vi "VI-Hacker v2.vi"(6 "Overwrite VI? (F)":bool, 8 "error in (no error)":errorcluster, 10 "Target Folder":path, 11 "VI Path":path) -> (0 "error out":errorcluster)   [LabVIEW 2020, in "VI-Hacker.lvlib"]
doc: "Unlocks a password protected VI.\n\nCreated by: Ryan Pacini (c) 2023"
uses:
  VI-Hacker.lvlib
panel:
  # "Unlock and Save Password Protected VI\nCreated by: Ryan Pacini (c) 2023"
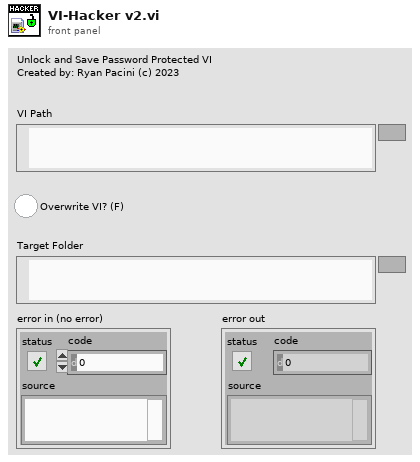
[diagram p1: front panel]
types:
  T1 = cluster{"BLOCK_INFO":cluster{"Int1":u32, "Int2":u32, "Int3":u32, "Offset":u32, "Size":u32}[]}
  T2 = cluster{"Name":string, "Idx":i32, "Data":string, "Offset":u32}
  T3 = enum16{"open", "replace", "create", "open or create", "replace or create", "replace or create with confirmation"}
  T4 = cluster{"vers":i32, "BDPW":i32, "LIBN":i32, "LVSR":i32, "BDHx":i32}
  T5 = cluster{"Version Major":u8, "Pswrd Hashes":cluster{"Pswrd (md5)":string, "Hash1 (md5)":string, "Hash2 (md5)":string}, "Owning Libs (':')":string, "Pswrd Salt (md5)":string, "Diagram (md5)":string, "BDPW Offset":u32, "New BDPW":string}
  T6 = cluster{"Pswrd (md5)":string, "Hash1 (md5)":string, "Hash2 (md5)":string}
  T7 = enum32{"invalid lock state", "Not Locked", "Locked (No Password)", "Password-protected"}
  T8 = cluster{"RSRC_Identifier":u64, "RSRC_Type":u32, "RSRC_Creator":u32, "Info_Offset":u32, "Info_Size":u32, "Data_Offset":u32, "Data_Size":u32}
  T9 = cluster{"Int1":u32, "Int2":u32, "Int3":u32, "Offset":u32, "Size":u32}
  T10 = cluster{"Int1":u32, "Int2":u32, "Int3":u32, "Offset":u32, "Size":u32}[]
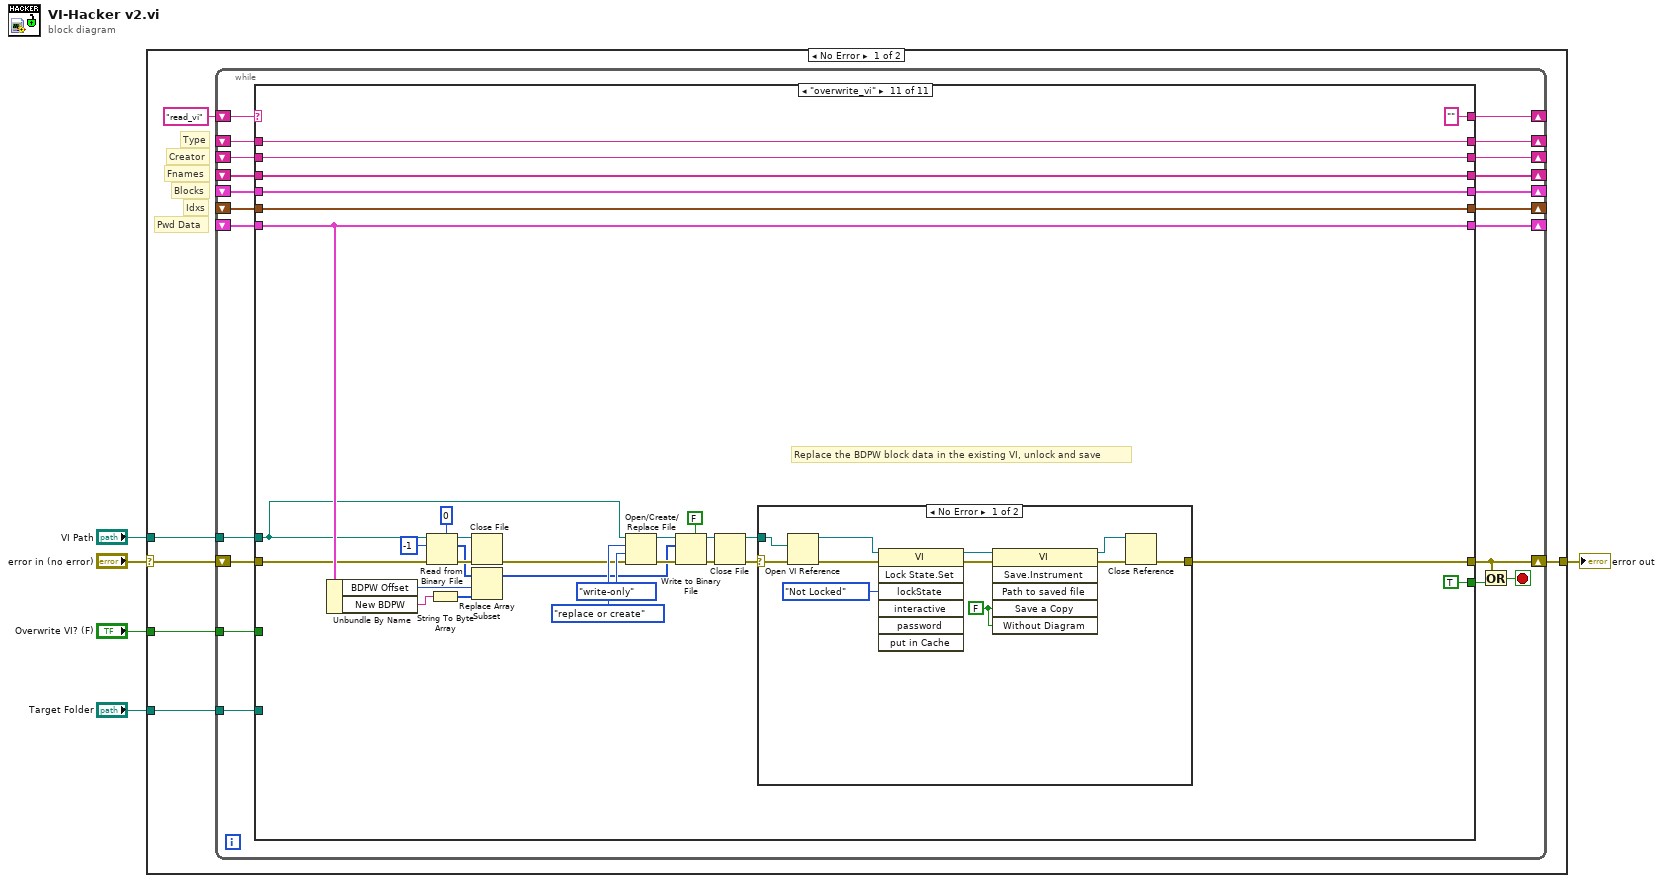
[diagram p0: block diagram]
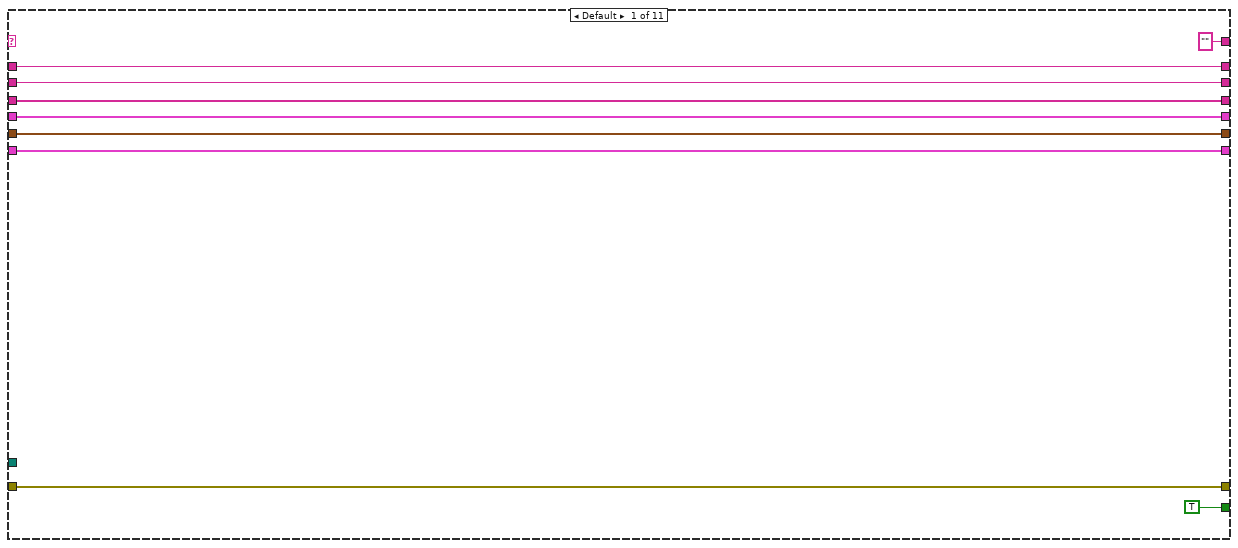
[diagram p2: hidden frame]
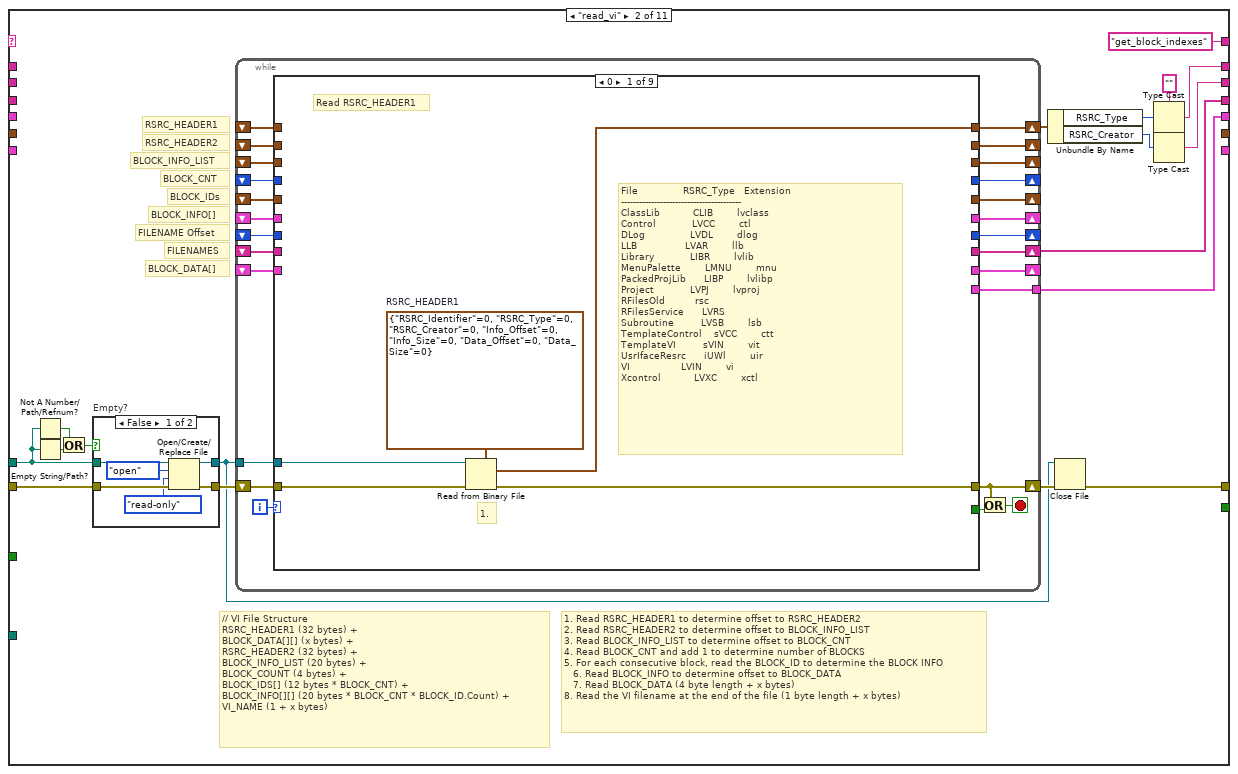
[diagram p3: hidden frame]
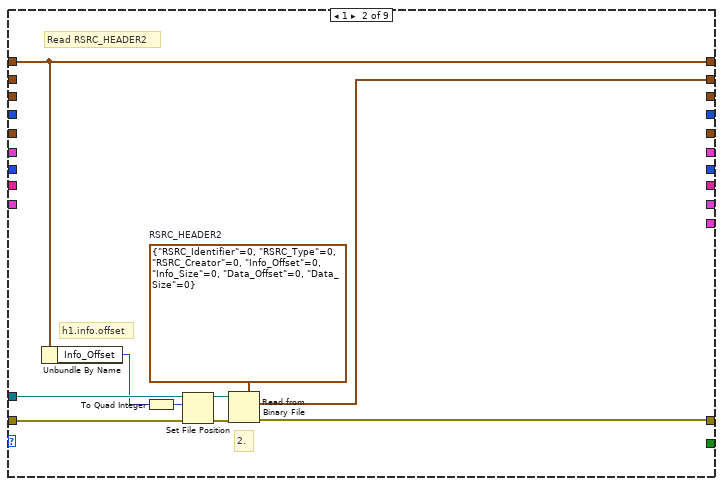
[diagram p4: hidden frame]
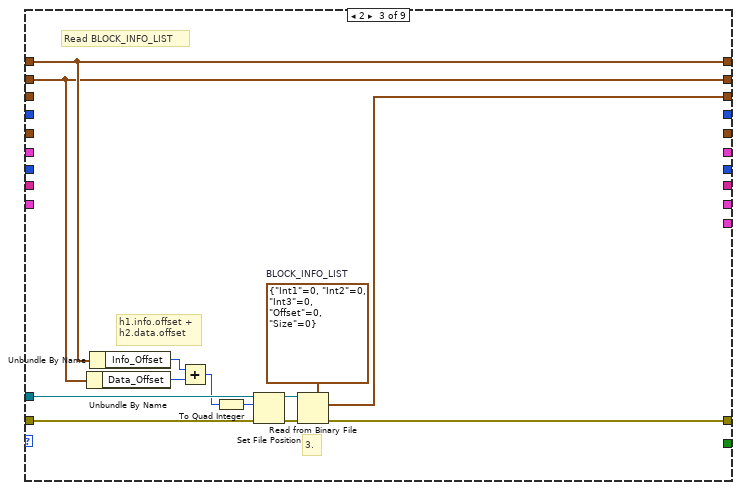
[diagram p5: hidden frame]
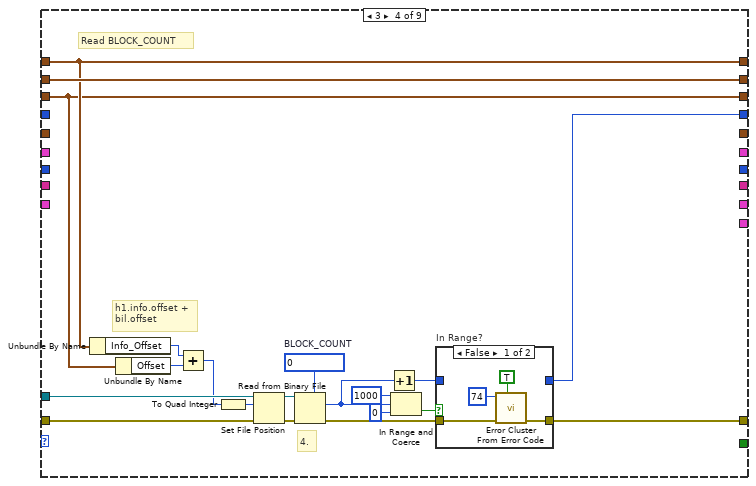
[diagram p6: hidden frame]
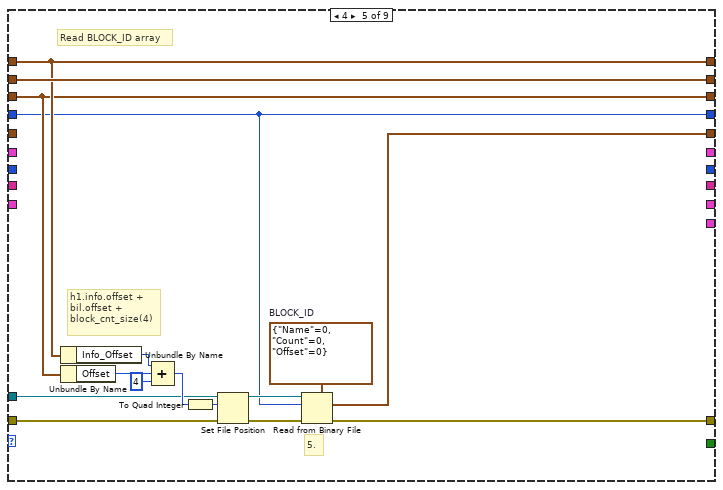
[diagram p8: hidden frame]
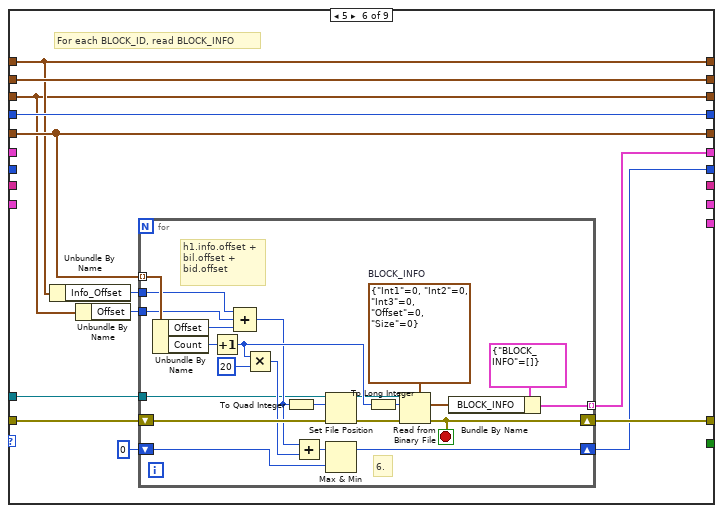
[diagram p9: hidden frame]
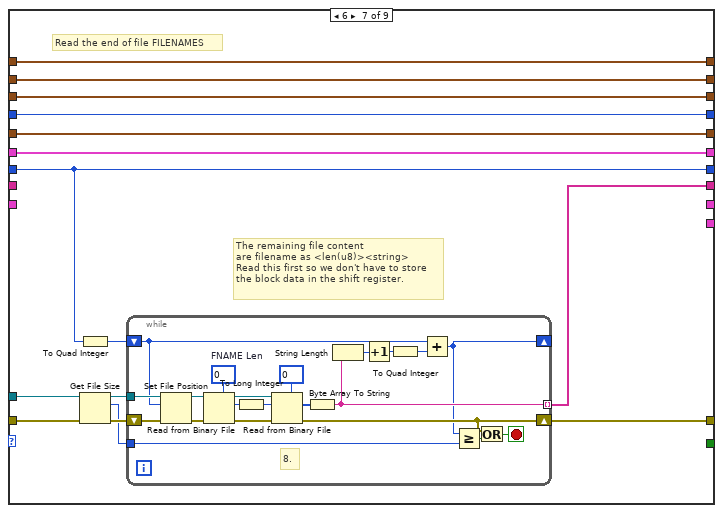
[diagram p10: hidden frame]
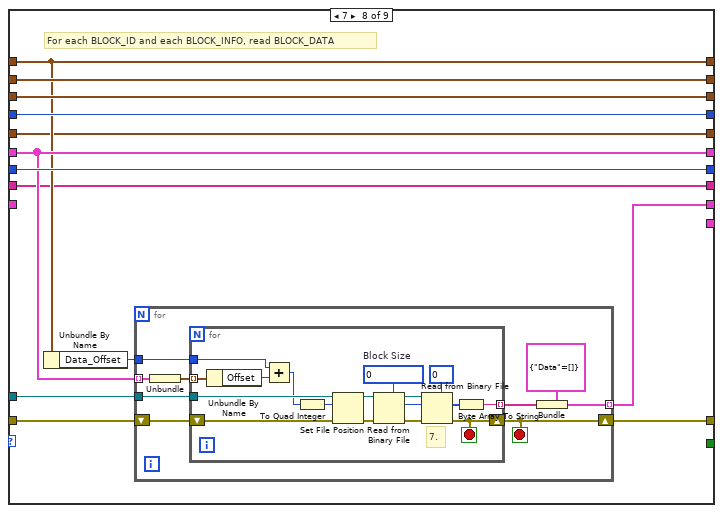
[diagram p11: hidden frame]
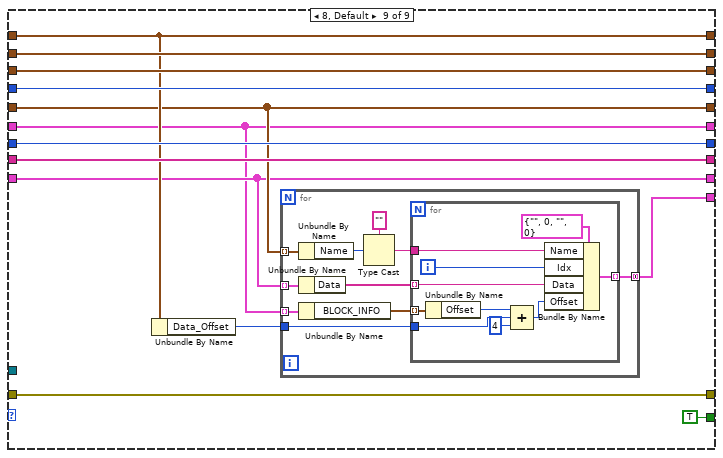
[diagram p12: hidden frame]
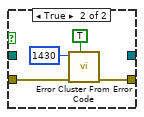
[diagram p13: hidden frame]
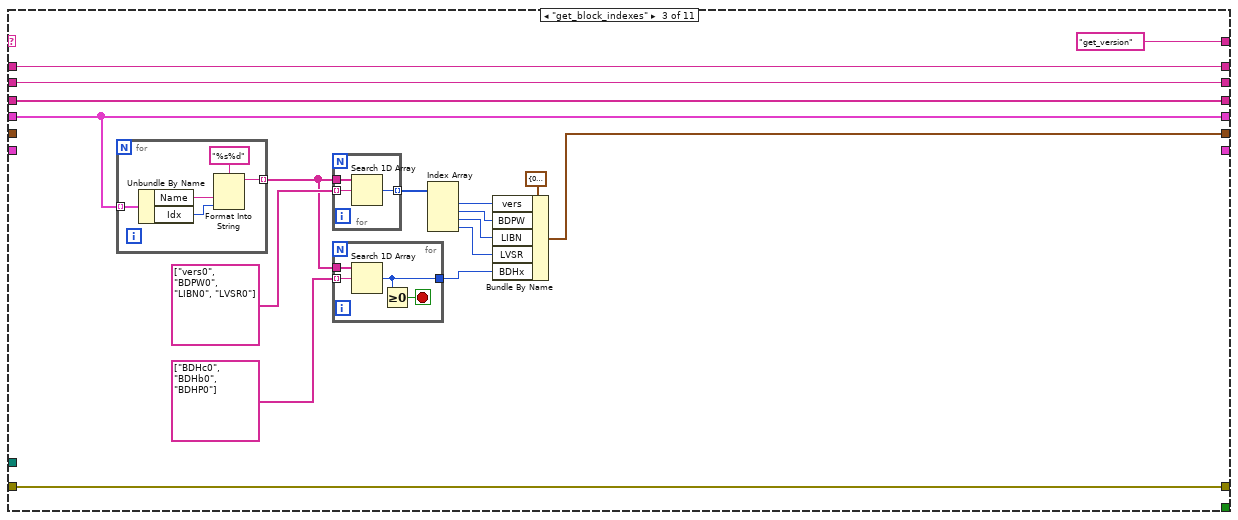
[diagram p14: hidden frame]
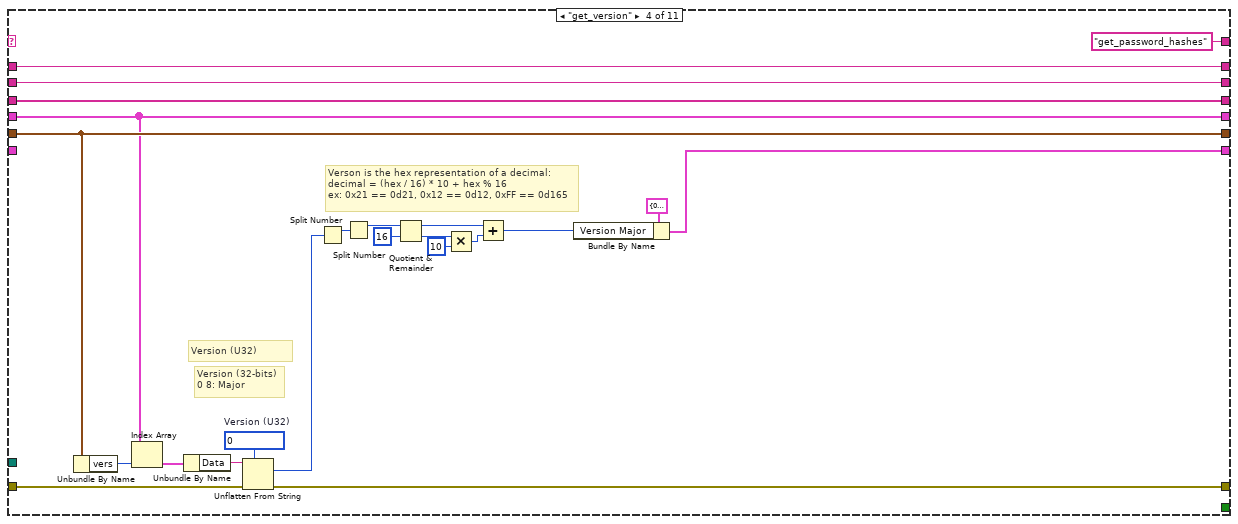
[diagram p15: hidden frame]
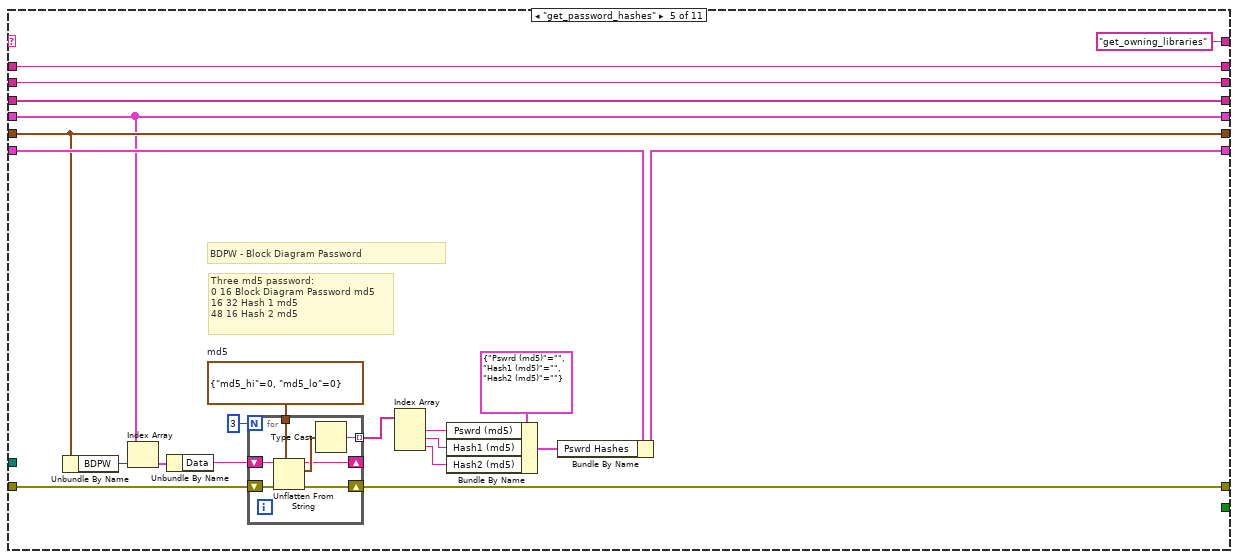
[diagram p16: hidden frame]
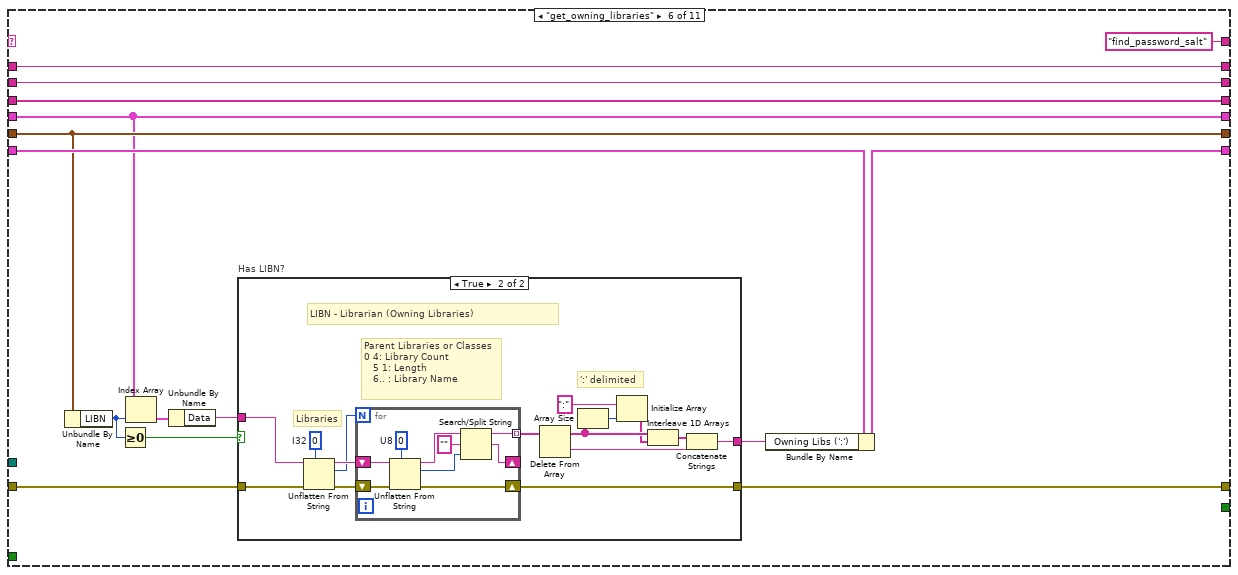
[diagram p17: hidden frame]
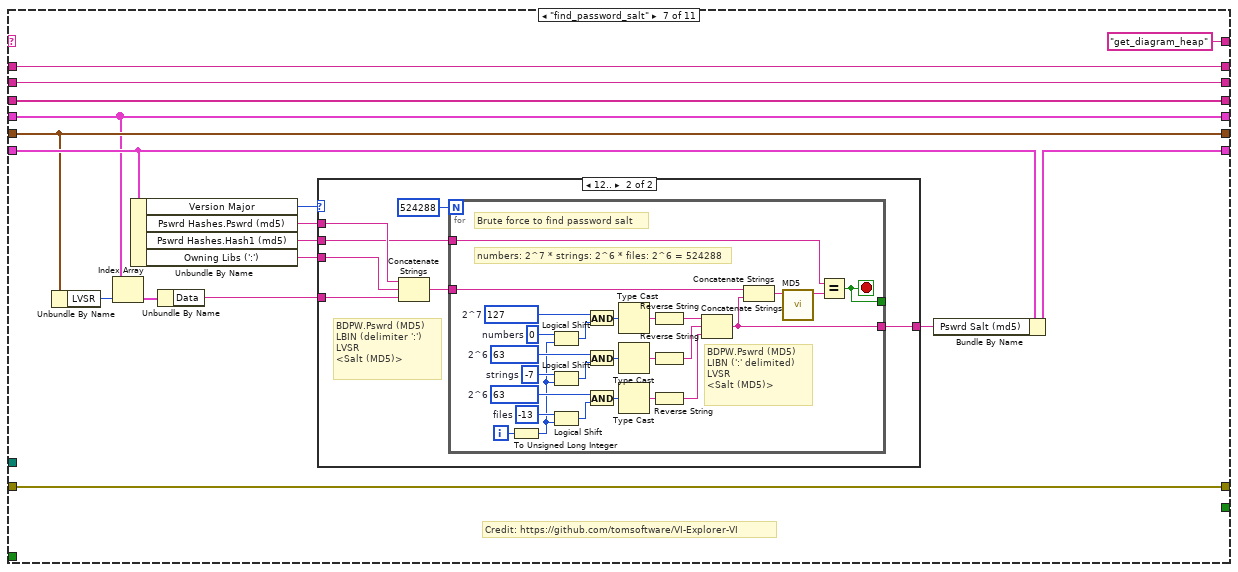
[diagram p19: hidden frame]
diagram:
  n1 = case shown="No Error" "error in (no error)" {
    selector: "error in (no error)" -> [w11 w639]
    tunnel: "VI Path" -> [w10 _]
    tunnel: [w9 w639] -> w4
    tunnel: "Target Folder" -> [w7 _]
    tunnel: "Overwrite VI? (F)" -> [w6 _]
    frame No Error {
      # "Pwd Data"
      # "Idxs"
      # "Blocks"
      # "Fnames"
      # "Creator"
      # "Type"
      n2 = while {
        tunnel: w10 -> [w31]
        shift-right: [w26] -> w9
        shift-left: w11 -> [w32]
        shift-right: [w24] -> _
        shift-left: "read_vi" -> [w27]
        shift-right: [w18] -> _
        shift-left: _ -> [w22]
        shift-right: [w30] -> _
        shift-left: _ -> [w21]
        shift-right: [w28] -> _
        shift-left: _ -> [w20]
        shift-right: [w29] -> _
        shift-left: _ -> [w19]
        shift-right: [w17] -> _
        shift-left: _ -> [w16]
        shift-right: [w15] -> _
        shift-left: _ -> [w14]
        tunnel: w7 -> [w13]
        tunnel: w6 -> [w12]
        stop <- w25 stop-if-true
        n3 = case shown="\"overwrite_vi\"" w27 {
          tunnel: w32 -> [w41 w59 w310 w341 w370 w394 w444 w486 w541 w546 w600]
          tunnel: w31 -> [_ w58 _ _ _ _ _ _ _ w543 w597]
          tunnel: [w38 w54 w325 w360 w381 w403 w445 w497 w542 w578 w626] -> w30
          tunnel: [w41 w51 w310 w340 w369 w393 w444 w483 w541 w547 w605] -> w26
          tunnel: [w39 w49 w322 w346 w366 w398 w435 w491 w524 w577 w625] -> w18
          tunnel: [w36 w45 w324 w359 w380 w402 w443 w496 w540 w576 w624] -> w29
          tunnel: [w37 w43 w323 w358 w379 w401 w442 w495 w539 w575 w623] -> w28
          tunnel: ["" "get_block_indexes" "get_version" "get_password_hashes" "get_owning_libraries" "find_password_salt" "get_diagram_heap" "calc_new_password" w513 "" ""] -> w24
          tunnel: [TRUE _ _ _ _ _ _ _ _ TRUE TRUE] -> w23
          tunnel: w22 -> [w39 _ w322 w346 w366 w398 w435 w491 w524 w577 w625]
          tunnel: w21 -> [w38 _ w325 w360 w381 w403 w445 w497 w542 w578 w626]
          tunnel: w20 -> [w37 _ w323 w358 w379 w401 w442 w495 w539 w575 w623]
          tunnel: w19 -> [w36 _ w324 w359 w380 w402 w443 w496 w540 w576 w624]
          tunnel: [w35 _ w311 w348 w368 w399 w437 w493 w526 w574 w622] -> w17
          tunnel: w16 -> [w35 _ _ w348 w368 w399 w437 w493 w526 w574 w622]
          tunnel: [w34 _ _ w339 w363 w396 w432 w481 w518 w550 w603] -> w15
          tunnel: w14 -> [w34 _ _ _ w378 w400 w439 w494 w530 w550 w603]
          tunnel: w13 -> [_ _ _ _ _ _ _ _ _ w544 _]
          tunnel: w12 -> [_ _ _ _ _ _ _ _ w514 _ _]
          frame Default {
          }
          frame "read_vi" {
            w42 = "" ("type")
            # "1. Read RSRC_HEADER1 to determine offset to RSRC_HEADER2\n2. Read RSRC_HEADER2 to determine offset to BLOCK_INFO_LIST\n3. Read BLOCK_INFO_LIST to determine offset to BLOCK_CNT\n4. Read BLOCK_CNT and add 1 to determine number of BLOCKS\n5. For each consecutive block, read the BLOCK_ID to determine the BLOCK INFO\n   6. Read BLOCK_INFO to determine offset to BLOCK_DATA\n   7. Read BLOCK_DATA (4 byte length + x bytes)\n8. Read the VI filename at the end of the file (1 byte length + x bytes)"
            # "// VI File Structure\nRSRC_HEADER1 (32 bytes) + \nBLOCK_DATA[][] (x bytes) +\nRSRC_HEADER2 (32 bytes) + \nBLOCK_INFO_LIST (20 bytes) +\nBLOCK_COUNT (4 bytes) + \nBLOCK_IDS[] (12 bytes * BLOCK_CNT) +\nBLOCK_INFO[][] (20 bytes * BLOCK_CNT * BLOCK_ID.Count) +\nVI_NAME (1 + x bytes)"
            # "BLOCK_DATA[]"
            # "FILENAME Offset"
            # "BLOCK_INFO[]"
            # "BLOCK_IDs"
            # "BLOCK_CNT"
            # "BLOCK_INFO_LIST"
            # "RSRC_HEADER2"
            # "FILENAMES"
            # "RSRC_HEADER1"
            n4 = Not A Number/Path/Refnum?(number/path/refnum=w58) -> (NaN/Path/Refnum?=w56:bool)
            n5 = Empty String/Path?(string/path=w58) -> (empty?=w57:bool)
            n6 = Or(x=w56, y=w57) -> (x .or. y?=w55:bool)
            n7 = case "Empty?" shown="False" w55 {
              tunnel: w59 -> [w304 w308]
              tunnel: w58 -> [w301 _]
              tunnel: [w300 w305] -> w53
              tunnel: [w299 _] -> w50
              frame False {
                n8 = Open/Create/Replace File(file path (use dialog)=w301, error in=w304, operation (0:open)=T3."open", access (0:read/write)=enum16{"read/write", "read-only", "write-only"}."read-only") -> (refnum out=w299:refnum<file>, error out=w300:errorcluster)  [unwired: 2 in, 1 out]
              }
              frame True {
                n9 = call <vilib>:"Error Cluster From Error Code.vi"("show call chain? (False)"=TRUE, "error in (no error)"=w308, "error code (0)"=1430) -> ("error out"=w305:errorcluster)  [unwired: 6 in]
              }
            }
            n10 = while {
              tunnel: w50 -> [w83]
              shift-right: [w79] -> w52
              shift-left: w53 -> [w84]
              shift-right: [w81] -> w48
              shift-left: _ -> [w80]
              shift-right: [w76] -> _
              shift-left: _ -> [w75]
              shift-right: [w74] -> _
              shift-left: _ -> [w73]
              shift-right: [w72] -> _
              shift-left: _ -> [w71]
              shift-right: [w70] -> _
              shift-left: _ -> [w69]
              shift-right: [w68] -> _
              shift-left: _ -> [w67]
              shift-right: [w66] -> _
              shift-left: _ -> [w65]
              shift-right: [w63] -> w54
              shift-left: _ -> [w62]
              shift-right: [w64] -> _
              shift-left: _ -> [w61]
              tunnel: [w60] -> w49
              i -> [w82]
              stop <- w78 stop-if-true
              n11 = case shown="0" w82 {
                tunnel: w84 -> [w89 w99 w112 w128 w151 w165 w199 w235 w272]
                tunnel: [w87 w97 w111 w127 w150 w163 w198 w229 w272] -> w79
                tunnel: w83 -> [w88 w94 w104 w117 w142 w164 w195 w231 _]
                tunnel: [w85 w98 w110 w126 w149 w161 w205 w233 w271] -> w81
                tunnel: w80 -> [_ w98 w110 w126 w149 w161 w205 w233 w271]
                tunnel: [_ _ _ _ _ _ _ _ TRUE] -> w77
                tunnel: [_ w96 w109 w132 w154 w167 w204 w239 w278] -> w76
                tunnel: w75 -> [_ _ w109 w132 w154 w167 w204 w239 w278]
                tunnel: [_ _ w106 w125 w148 w160 w203 w238 w277] -> w74
                tunnel: w73 -> [_ _ _ w125 w148 w160 w203 w238 w277]
                tunnel: [_ _ _ w119 w140 w166 w202 w237 w276] -> w72
                tunnel: w71 -> [_ _ _ _ w140 w166 w202 w237 w276]
                tunnel: [_ _ _ _ w139 w162 w201 w230 w270] -> w70
                tunnel: w69 -> [_ _ _ _ _ w162 w201 w230 w270]
                tunnel: [_ _ _ _ _ w156 w200 w234 w267] -> w68
                tunnel: w67 -> [_ _ _ _ _ _ w200 w234 w267]
                tunnel: [_ _ _ _ _ w155 w193 w236 w275] -> w66
                tunnel: w65 -> [_ _ _ _ _ _ w193 w236 w275]
                tunnel: [_ _ _ _ _ _ _ w228 w269] -> w64
                tunnel: [_ _ _ _ _ _ w197 w227 w274] -> w63
                tunnel: w62 -> [_ _ _ _ _ _ _ w227 w274]
                tunnel: w61 -> [_ _ _ _ _ _ _ _ w269]
                tunnel: [_ _ _ _ _ _ _ _ w268] -> w60
                frame 0 {
                  w86 = T8 {"RSRC_Identifier"=0, "RSRC_Type"=0, "RSRC_Creator"=0, "Info_Offset"=0, "Info_Size"=0, "Data_Offset"=0, "Data_Size"=0}  # RSRC_HEADER1
                  # "File               RSRC_Type   Extension\n----------------------------------------\nClassLib           CLIB        lvclass\nControl            LVCC        ctl\nDLog               LVDL        dlog\nLLB                LVAR        llb\nLibrary            LIBR        lvlib\nMenuPalette        LMNU        mnu\nPackedProjLib      LIBP        lvlibp\nProject            LVPJ        lvproj\nRFilesOld          rsc         \nRFilesService      LVRS        \nSubroutine         LVSB        lsb\nTemplateControl    sVCC        ctt\nTemplateVI         sVIN        vit\nUsrIfaceResrc      iUWl        uir\nVI                 LVIN        vi\nXcontrol           LVXC        xctl"
                  # "Read RSRC_HEADER1"
                  # "1."
                  n12 = Read from Binary File(5:w86, 8:w89, 11:w88) -> (0:w87:errorcluster, 2:w85:T8)  [unwired: 3 in, 2 out]
                }
                frame 1 {
                  w92 = T8 {"RSRC_Identifier"=0, "RSRC_Type"=0, "RSRC_Creator"=0, "Info_Offset"=0, "Info_Size"=0, "Data_Offset"=0, "Data_Size"=0}  # RSRC_HEADER2
                  # "Read RSRC_HEADER2"
                  # "2."
                  # "h1.info.offset"
                  n13 = Unbundle By Name(w98) -> ("Info_Offset"=w93:u32)
                  n14 = To Quad Integer(1:w93) -> (0:w90:i64)
                  n15 = Set File Position(offset (in bytes) (0)=w90, refnum=w94, error in=w99) -> (refnum out=w91:refnum<file>, error out=w95:errorcluster)  [unwired: 1 in]
                  n16 = Read from Binary File(5:w92, 8:w95, 11:w91) -> (0:w97:errorcluster, 2:w96:T8)  [unwired: 3 in, 2 out]
                }
                frame 2 {
                  w103 = T9 {"Int1"=0, "Int2"=0, "Int3"=0, "Offset"=0, "Size"=0}  # BLOCK_INFO_LIST
                  # "Read BLOCK_INFO_LIST"
                  # "3."
                  # "h1.info.offset +\nh2.data.offset"
                  n17 = Unbundle By Name(w109) -> ("Data_Offset"=w108:u32)
                  n18 = Unbundle By Name(w110) -> ("Info_Offset"=w107:u32)
                  n19 = Add(x=w107, y=w108) -> (x+y=w101:u32)
                  n20 = To Quad Integer(1:w101) -> (0:w100:i64)
                  n21 = Set File Position(offset (in bytes) (0)=w100, refnum=w104, error in=w112) -> (refnum out=w102:refnum<file>, error out=w105:errorcluster)  [unwired: 1 in]
                  n22 = Read from Binary File(5:w103, 8:w105, 11:w102) -> (0:w111:errorcluster, 2:w106:T9)  [unwired: 3 in, 2 out]
                }
                frame 3 {
                  w116 = 0  # BLOCK_COUNT
                  # "Read BLOCK_COUNT"
                  # "4."
                  # "h1.info.offset +\nbil.offset"
                  n23 = Unbundle By Name(w126) -> ("Info_Offset"=w123:u32)
                  n24 = Unbundle By Name(w125) -> ("Offset"=w124:u32)
                  n25 = Add(x=w123, y=w124) -> (x+y=w114:u32)
                  n26 = To Quad Integer(1:w114) -> (0:w113:i64)
                  n27 = Set File Position(offset (in bytes) (0)=w113, refnum=w117, error in=w128) -> (refnum out=w115:refnum<file>, error out=w118:errorcluster)  [unwired: 1 in]
                  n28 = Read from Binary File(5:w116, 8:w118, 11:w115) -> (0:w129:errorcluster, 2:w120:i32)  [unwired: 3 in, 2 out]
                  n29 = Increment(x=w120) -> (x+1=w121:i32)
                  n30 = In Range and Coerce(upper limit=1000, x=w120, lower limit=0) -> (In Range?=w122:bool)  [unwired: 1 out]
                  n31 = case "In Range?" shown="False" w122 {
                    tunnel: w129 -> [w134 w138]
                    tunnel: [w133 w138] -> w127
                    tunnel: w121 -> [_ w137]
                    tunnel: [_ w137] -> w119
                    frame False {
                      n32 = call <vilib>:"Error Cluster From Error Code.vi"("show call chain? (False)"=TRUE, "error in (no error)"=w134, "error code (0)"=74) -> ("error out"=w133:errorcluster)  [unwired: 6 in]
                    }
                    frame True {
                    }
                  }
                }
                frame 4 {
                  w144 = cluster{"Name":u32, "Count":u32, "Offset":u32} {"Name"=0, "Count"=0, "Offset"=0}  # BLOCK_ID
                  # "Read BLOCK_ID array"
                  # "5."
                  # "h1.info.offset +\nbil.offset +\nblock_cnt_size(4)"
                  n33 = Unbundle By Name(w149) -> ("Info_Offset"=w153:u32)
                  n34 = Unbundle By Name(w148) -> ("Offset"=w152:u32)
                  n35 = Compound Arithmetic op=ADD(w153, w152, u32 4 ("value")) -> (w143:u32)
                  n36 = To Quad Integer(1:w143) -> (0:w141:i64)
                  n37 = Set File Position(offset (in bytes) (0)=w141, refnum=w142, error in=w151) -> (refnum out=w145:refnum<file>, error out=w146:errorcluster)  [unwired: 1 in]
                  n38 = Read from Binary File(5:w144, 8:w146, 10:w140, 11:w145) -> (0:w150:errorcluster, 2:w139:cluster{"Name":u32, "Count":u32, "Offset":u32}[])  [unwired: 2 in, 2 out]
                }
                frame 5 {
                  # "For each BLOCK_ID, read BLOCK_INFO"
                  n39 = Unbundle By Name(w161) -> ("Info_Offset"=w159:u32)
                  n40 = Unbundle By Name(w160) -> ("Offset"=w158:u32)
                  n41 = for {
                    tunnel: w164 -> [w170]
                    shift-right: [w177] -> w163
                    shift-left: w165 -> [w190]
                    tunnel: w162 -> [w189] mode=indexing
                    tunnel: w159 -> [w185]
                    tunnel: w158 -> [w184]
                    shift-right: [w181] -> w155
                    shift-left: u32 0 -> [w180]
                    tunnel: [w178] -> w156 mode=indexing
                    stop <- w177 stop-if-true
                    w176 = T9 {"Int1"=0, "Int2"=0, "Int3"=0, "Offset"=0, "Size"=0}  # BLOCK_INFO
                    # "6."
                    # "h1.info.offset +\nbil.offset +\nbid.offset"
                    n42 = Unbundle By Name(w189) -> ("Offset"=w186:u32, "Count"=w187:u32)
                    n43 = Increment(x=w187) -> (x+1=w175:u32)
                    n44 = Compound Arithmetic op=ADD(w185, w184, w186) -> (w171:u32)
                    n45 = Multiply(x=w175, y=u32 20 ("length (rest)")) -> (x*y=w183:u32)
                    n46 = To Quad Integer(1:w171) -> (0:w169:i64)
                    n47 = Add(x=w171, y=w183) -> (x+y=w182:u32)
                    n48 = Set File Position(offset (in bytes) (0)=w169, refnum=w170, error in=w190) -> (refnum out=w173:refnum<file>, error out=w174:errorcluster)  [unwired: 1 in]
                    n49 = Max & Min(x=w182, y=w180) -> (max(x,y)=w181:u32)  [unwired: 1 out]
                    n50 = To Long Integer(number=w175) -> (32bit integer=w172:i32)
                    n51 = Read from Binary File(5:w176, 8:w174, 10:w172, 11:w173) -> (0:w177:errorcluster, 2:w179:T10)  [unwired: 2 in, 2 out]
                    n52 = Bundle By Name(cluster=T1 {"BLOCK_INFO"=[]}, "BLOCK_INFO"=w179) -> (w178:T1)
                  }
                }
                frame 6 {
                  # "Read the end of file FILENAMES"
                  # "The remaining file content\nare filename as <len(u8)><string>\nRead this first so we don't have to store\nthe block data in the shift register."
                  n53 = To Quad Integer(1:w193) -> (0:w192:i64)
                  n54 = Get File Size(file=w195, error in=w199) -> (refnum out=w194:refnum<file>, size (in bytes)=w191:i64, 0:w196:errorcluster)
                  n55 = while {
                    tunnel: [w215] -> w197 mode=indexing
                    tunnel: w194 -> [w224]
                    shift-right: [w213] -> w198
                    shift-left: w196 -> [w226]
                    shift-right: [w208] -> _
                    shift-left: w192 -> [w209]
                    tunnel: w191 -> [w207]
                    stop <- w212 stop-if-true
                    w221 = u8 0  # FNAME Len
                    # "8."
                    n56 = Set File Position(offset (in bytes) (0)=w209, refnum=w224, error in=w226) -> (refnum out=w223:refnum<file>, error out=w225:errorcluster)  [unwired: 1 in]
                    n57 = Read from Binary File(5:w221, 8:w225, 11:w223) -> (0:w222:errorcluster, 2:w218:u8, 3:w219:refnum<file>)  [unwired: 3 in, 1 out]
                    n58 = To Long Integer(number=w218) -> (32bit integer=w217:i32)
                    n59 = Read from Binary File(5:u8 0, 8:w222, 10:w217, 11:w219) -> (0:w213:errorcluster, 2:w216:u8[])  [unwired: 2 in, 2 out]
                    n60 = Byte Array To String(unsigned byte array=w216) -> (string=w215:string)
                    n61 = String Length(string=w215) -> (length=w214:i32)
                    n62 = Increment(x=w214) -> (x+1=w211:i32)
                    n63 = To Quad Integer(1:w211) -> (0:w210:i64)
                    n64 = Add(x=w209, y=w210) -> (x+y=w208:i64)
                    n65 = Greater Or Equal?(x=w208, y=w207) -> (x >= y?=w206:bool)
                    n66 = Or(x=w213, y=w206) -> (x .or. y?=w212:bool)
                  }
                }
                frame 7 {
                  # "For each BLOCK_ID and each BLOCK_INFO, read BLOCK_DATA"
                  n67 = Unbundle By Name(w233) -> ("Data_Offset"=w232:u32)
                  n68 = for {
                    tunnel: w234 -> [w247] mode=indexing
                    tunnel: w232 -> [w245]
                    tunnel: w231 -> [w244]
                    shift-right: [w243] -> w229
                    shift-left: w235 -> [w248]
                    tunnel: [w241] -> w228 mode=indexing
                    stop <- w243 stop-if-true
                    n69 = Unbundle(w247) -> ("BLOCK_INFO"=w246:T10)
                    n70 = for {
                      tunnel: w244 -> [w258]
                      shift-right: [w260] -> w243
                      shift-left: w248 -> [w265]
                      tunnel: [w249] -> w242 mode=indexing
                      tunnel: w246 -> [w262] mode=indexing
                      tunnel: w245 -> [w261]
                      stop <- w260 stop-if-true
                      w252 = 0  # Block Size
                      # "7."
                      n71 = Unbundle By Name(w262) -> ("Offset"=w264:u32)
                      n72 = Add(x=w261, y=w264) -> (x+y=w257:u32)
                      n73 = To Quad Integer(1:w257) -> (0:w256:i64)
                      n74 = Set File Position(offset (in bytes) (0)=w256, refnum=w258, error in=w265) -> (refnum out=w254:refnum<file>, error out=w259:errorcluster)  [unwired: 1 in]
                      n75 = Read from Binary File(5:w252, 8:w259, 11:w254) -> (0:w255:errorcluster, 2:w250:i32, 3:w253:refnum<file>)  [unwired: 3 in, 1 out]
                      n76 = Read from Binary File(5:u8 0, 8:w255, 10:w250, 11:w253) -> (0:w260:errorcluster, 2:w263:u8[])  [unwired: 2 in, 2 out]
                      n77 = Byte Array To String(unsigned byte array=w263) -> (string=w249:string)
                    }
                    n78 = Bundle(cluster=cluster{"Data":string[]} {"Data"=[]}, "Data"=w242) -> (w241:cluster{"Data":string[]})
                  }
                }
                frame 8, Default {
                  n79 = Unbundle By Name(w271) -> ("Data_Offset"=w266:u32)
                  n80 = for {
                    tunnel: w270 -> [w288] mode=indexing
                    tunnel: [w279] -> w268 mode=concatenating
                    tunnel: w269 -> [w285] mode=indexing
                    tunnel: w267 -> [w284] mode=indexing
                    tunnel: w266 -> [w282]
                    n81 = Unbundle By Name(w288) -> ("Name"=w287:u32)
                    n82 = Unbundle By Name(w285) -> ("Data"=w281:string[])
                    n83 = Unbundle By Name(w284) -> ("BLOCK_INFO"=w283:T10)
                    n84 = Type Cast(type="", x=w287) -> (*(type *) &x=w280:string)
                    n85 = for {
                      tunnel: w283 -> [w298] mode=indexing
                      tunnel: w282 -> [w296]
                      tunnel: w281 -> [w291] mode=indexing
                      tunnel: w280 -> [w293]
                      tunnel: [w289] -> w279 mode=indexing
                      i -> [w292]
                      n86 = Unbundle By Name(w298) -> ("Offset"=w295:u32)
                      n87 = Compound Arithmetic op=ADD(w295, w296, u32 4 ("value")) -> (w290:u32)
                      n88 = Bundle By Name(cluster=T2 {"Name"="", "Idx"=0, "Data"="", "Offset"=0} ("Block"), "Name"=w293, "Idx"=w292, "Data"=w291, "Offset"=w290) -> (w289:T2)
                    }
                  }
                }
              }
              n89 = Or(x=w79, y=w77) -> (x .or. y?=w78:bool)
            }
            n90 = Unbundle By Name(w48) -> ("RSRC_Type"=w47:u32, "RSRC_Creator"=w46:u32)
            n91 = Close File(refnum=w50, error in=w52) -> (error out=w51:errorcluster)  [unwired: 1 out]
            n92 = Type Cast(type=w42, x=w47) -> (*(type *) &x=w45:string)
            n93 = Type Cast(type=w42, x=w46) -> (*(type *) &x=w43:string)
          }
          frame "get_block_indexes" {
            n94 = for {
              tunnel: w322 -> [w337] mode=indexing
              tunnel: [w333] -> w314 mode=indexing
              n95 = Unbundle By Name(w337) -> ("Name"=w336:string, "Idx"=w334:i32)
              n96 = Format Into String(format string="%s%d", w336, w334) -> (resulting string=w333:string)  [unwired: 2 in, 1 out]
            }
            n97 = for {
              tunnel: w314 -> [w332]
              tunnel: string[] ["vers0", "BDPW0", "LIBN0", "LVSR0"] -> [w331] mode=indexing
              tunnel: [w330] -> w320 mode=indexing
              n98 = Search 1D Array(1D array=w332, element=w331) -> (index of element=w330:i32)  [unwired: 1 in]
            }
            n99 = for {
              tunnel: w314 -> [w329]
              tunnel: string[] ["BDHc0", "BDHb0", "BDHP0"] -> [w328] mode=indexing
              tunnel: [w327] -> w312
              stop <- w326 stop-if-true
              n100 = Search 1D Array(1D array=w329, element=w328) -> (index of element=w327:i32)  [unwired: 1 in]
              n101 = Greater Or Equal To 0?(x=w327) -> (x >= 0?=w326:bool)
            }
            n102 = Index Array(array=w320) -> (element #1=w318:i32, element #2=w317:i32, element #3=w316:i32, element #4=w315:i32)  [unwired: 4 in]
            n103 = Bundle By Name(cluster=T4 {"vers"=0, "BDPW"=0, "LIBN"=0, "LVSR"=0, "BDHx"=0} ("Block Idxs"), "vers"=w318, "BDPW"=w317, "LIBN"=w316, "LVSR"=w315, "BDHx"=w312) -> (w311:T4)
          }
          frame "get_version" {
            w350 = u32 0  # Version (U32)
            # "Version (U32)"
            # "Verson is the hex representation of a decimal:\ndecimal = (hex / 16) * 10 + hex % 16\nex: 0x21 == 0d21, 0x12 == 0d12, 0xFF == 0d165"
            # "Version (32-bits)\n0 8: Major"
            n104 = Unbundle By Name(w348) -> ("vers"=w347:i32)
            n105 = Index Array(array=w346, index=w347) -> (element=w345:T2)
            n106 = Unbundle By Name(w345) -> ("Data"=w344:string)
            n107 = Unflatten From String(type=w350, binary string=w344, error in (no error)=w341) -> (value=w349:u32, error out=w340:errorcluster)  [unwired: 2 in, 1 out]
            n108 = Split Number(x=w349) -> (hi(x)=w357:u16)  [unwired: 1 out]
            n109 = Split Number(x=w357) -> (hi(x)=w356:u8)  [unwired: 1 out]
            n110 = Quotient & Remainder(x=w356, y=u8 16) -> (x-y*floor(x/y)=w351:u8, floor(x/y)=w354:u8)
            n111 = Multiply(x=w354, y=u8 10) -> (x*y=w352:u8)
            n112 = Add(x=w351, y=w352) -> (x+y=w342:u8)
            n113 = Bundle By Name(cluster=T5 {"Version Major"=0, "Pswrd Hashes"={"Pswrd (md5)"="", "Hash1 (md5)"="", "Hash2 (md5)"=""}, "Owning Libs (':')"="", "Pswrd Salt (md5)"="", "Diagram (md5)"="", "BDPW Offset"=0, "New BDPW"=""} ("Pwd"), "Version Major"=w342) -> (w339:T5)
          }
          frame "get_password_hashes" {
            w372 = cluster{"md5_hi":u64, "md5_lo":u64} {"md5_hi"=0, "md5_lo"=0}  # md5
            # "BDPW - Block Diagram Password"
            # "Three md5 password:\n0 16 Block Diagram Password md5\n16 32 Hash 1 md5\n48 16 Hash 2 md5"
            n114 = Unbundle By Name(w368) -> ("BDPW"=w367:i32)
            n115 = Index Array(array=w366, index=w367) -> (element=w365:T2)
            n116 = Unbundle By Name(w365) -> ("Data"=w364:string)
            n117 = for {
              N: 3 -> [_]
              shift-right: [w388] -> w369
              shift-left: w370 -> [w387]
              tunnel: [w384] -> w376 mode=indexing
              shift-right: [w383] -> _
              shift-left: w364 -> [w386]
              tunnel: w372 -> [w382]
              n118 = Unflatten From String(type=w382, binary string=w386, error in (no error)=w387) -> (rest of the binary string=w383:string, value=w385:cluster{"md5_hi":u64, "md5_lo":u64}, error out=w388:errorcluster)  [unwired: 2 in]
              n119 = Type Cast(x=w385) -> (*(type *) &x=w384:string)  [unwired: 1 in]
            }
            n120 = Index Array(array=w376) -> (element #1=w375:string, element #2=w374:string, element #3=w373:string)  [unwired: 3 in]
            n121 = Bundle By Name(cluster=T6 {"Pswrd (md5)"="", "Hash1 (md5)"="", "Hash2 (md5)"=""} ("BDPW"), "Pswrd (md5)"=w375, "Hash1 (md5)"=w374, "Hash2 (md5)"=w373) -> (w362:T6)
            n122 = Bundle By Name(cluster=w378, "Pswrd Hashes"=w362) -> (w363:T5)
          }
          frame "get_owning_libraries" {
            n123 = Unbundle By Name(w399) -> ("LIBN"=w390:i32)
            n124 = Greater Or Equal To 0?(x=w390) -> (x >= 0?=w389:bool)
            n125 = Index Array(array=w398, index=w390) -> (element=w397:T2)
            n126 = Unbundle By Name(w397) -> ("Data"=w392:string)
            n127 = case "Has LIBN?" shown="True" w389 {
              tunnel: w394 -> [w404 w408]
              tunnel: [w404 w407] -> w393
              tunnel: w392 -> [_ w406]
              tunnel: [_ w405] -> w391
              frame False {
              }
              frame True {
                w419 = 0  # I32
                # "':' delimited"
                # "LIBN - Librarian (Owning Libraries)"
                # "Parent Libraries or Classes\n0 4: Library Count\n   5 1: Length\n   6.. : Library Name"
                # "Libraries"
                n128 = Unflatten From String(type=w419, binary string=w406, error in (no error)=w408) -> (rest of the binary string=w417:string, value=w416:i32, error out=w418:errorcluster)  [unwired: 2 in]
                n129 = for {
                  N: w416 -> [_]
                  shift-right: [w421] -> _
                  shift-left: w417 -> [w426]
                  shift-right: [w422] -> w407
                  shift-left: w418 -> [w427]
                  tunnel: [w420] -> w409 mode=indexing
                  w428 = u8 0  # U8
                  n130 = Unflatten From String(type=w428, binary string=w426, error in (no error)=w427) -> (rest of the binary string=w425:string, value=w424:u8, error out=w422:errorcluster)  [unwired: 2 in]
                  n131 = Search/Split String(string=w425, search string/char (-)="", offset (0)=w424) -> (substring before match=w420:string, match + rest of string=w421:string)  [unwired: 1 out]
                }
                n132 = Delete From Array(array=w409) -> (deleted portion=w410:string, array with subset deleted=w413:string[])  [unwired: 2 in]
                n133 = Array Size(array=w413) -> (size(s)=w415:i32)
                n134 = Initialize Array(":", w415) -> (w412:string[])
                n135 = Interleave 1D Arrays(w413, w412) -> (w411:string[])
                n136 = Concatenate Strings(w411, w410) -> (w405:string)
              }
            }
            n137 = Bundle By Name(cluster=w400, "Owning Libs (':')"=w391) -> (w396:T5)
          }
          frame "find_password_salt" {
            # "Credit: https://github.com/tomsoftware/VI-Explorer-VI"
            n138 = Unbundle By Name(w437) -> ("LVSR"=w436:i32)
            n139 = Index Array(array=w435, index=w436) -> (element=w434:T2)
            n140 = Unbundle By Name(w439) -> ("Version Major"=w431:u8, "Pswrd Hashes.Pswrd (md5)"=w441:string, "Pswrd Hashes.Hash1 (md5)"=w440:string, "Owning Libs (':')"=w438:string)
            n141 = Unbundle By Name(w434) -> ("Data"=w433:string)
            n142 = case shown="12.." w431 {
              tunnel: w441 -> [_ w450]
              tunnel: w440 -> [_ w449]
              tunnel: w438 -> [_ w448]
              tunnel: w433 -> [_ w447]
              tunnel: [_ w446] -> w430
              frame ..11 {
              }
              frame 12.. {
                # "BDPW.Pswrd (MD5)\nLBIN (delimiter ':')\nLVSR\n<Salt (MD5)>"
                n143 = Concatenate Strings(w450, w448, w447) -> (w451:string)
                n144 = for {
                  N: 524288 -> [_]
                  tunnel: w451 -> [w478]
                  tunnel: w449 -> [w477]
                  tunnel: [w468] -> _
                  tunnel: [w455] -> w446
                  i -> [w473]
                  stop <- w468 stop-if-true
                  w466 = u32 63  # 2^6
                  w467 = u32 63  # 2^6
                  w470 = i8 -13  # files
                  w471 = i8 -7  # strings
                  w472 = i8 0  # numbers
                  w469 = u32 127  # 2^7
                  # "numbers: 2^7 * strings: 2^6 * files: 2^6 = 524288"
                  # "BDPW.Pswrd (MD5)\nLIBN (':' delimited)\nLVSR\n<Salt (MD5)>"
                  # "Brute force to find password salt"
                  n145 = To Unsigned Long Integer(number=w473) -> (unsigned 32bit integer=w465:u32)
                  n146 = Logical Shift(y=w472, x=w465) -> (x << y=w476:u32)
                  n147 = Logical Shift(y=w471, x=w465) -> (x << y=w474:u32)
                  n148 = Logical Shift(y=w470, x=w465) -> (x << y=w475:u32)
                  n149 = And(x=w469, y=w476) -> (x .and. y?=w461:u32)
                  n150 = And(x=w466, y=w474) -> (x .and. y?=w460:u32)
                  n151 = And(x=w467, y=w475) -> (x .and. y?=w459:u32)
                  n152 = Type Cast(x=w461) -> (*(type *) &x=w464:string)  [unwired: 1 in]
                  n153 = Type Cast(x=w460) -> (*(type *) &x=w463:string)  [unwired: 1 in]
                  n154 = Type Cast(x=w459) -> (*(type *) &x=w462:string)  [unwired: 1 in]
                  n155 = Reverse String(1:w464) -> (0:w458:string)
                  n156 = Reverse String(1:w463) -> (0:w457:string)
                  n157 = Reverse String(1:w462) -> (0:w456:string)
                  n158 = Concatenate Strings(w458, w457, w456) -> (w455:string)
                  n159 = Concatenate Strings(w478, w455) -> (w454:string)
                  n160 = call "MD5.vi"("Message String"=w454) -> ("MD5 (16-bytes)"=w453:string)  [unwired: 9 in, 1 out]
                  n161 = Equal?(x=w477, y=w453) -> (x = y?=w468:bool)
                }
              }
            }
            n162 = Bundle By Name(cluster=w439, "Pswrd Salt (md5)"=w430) -> (w432:T5)
          }
          frame "get_diagram_heap" {
            # "Diagram (md5)"
            # "BDHP, BDHb, BDHc - Block Diagram Heap (Source Code)\nFPHP, FPHb, FPHc - Front Panel Heap (Source Code)"
            # "Block Diagram/Front Panel Heap (LabVIEW Version .. 5)\nBlock Diagram/Front Panel Heap Version B (LabVIEW Version 6 .. 9) - Compressed using deflate\nBlock Diagram/Front Panel Heap Version C (LabVIEW Version 10 .. 22) - Compressed using deflate"
            n163 = Unbundle By Name(w493) -> ("BDHx"=w492:i32)
            n164 = Index Array(array=w491, index=w492) -> (element=w490:T2)
            n165 = Unbundle By Name(w490) -> ("Name"=w484:string, "Data"=w485:string)
            n166 = Equal?(x=string[] ["BDHb", "BDHc", "FPHb", "FPHc"], y=w484) -> (x = y?=w488:bool[])
            n167 = Or Array Elements(Boolean array=w488) -> (logical OR=w487:bool)
            n168 = case "Is Compressed?" shown="True" w487 {
              tunnel: w485 -> [w499 w511]
              tunnel: w486 -> [w498 w506]
              tunnel: [w498 w502] -> w483
              tunnel: [w499 w500] -> w482
              frame False {
              }
              frame True {
                w508 = u32 0  # Uncompressed Size
                n169 = Unflatten From String(type=w508, binary string=w511, error in (no error)=w506) -> (rest of the binary string=w510:string, value=w507:u32, error out=w509:errorcluster)  [unwired: 2 in]
                n170 = call "zlib Uncompress.vi"("error in (no error)"=w509, "Uncompressed Size in"=w507, "Compressed Data in"=w510) -> ("error out"=w503:errorcluster, "Uncompressed Data out"=w501:string)  [unwired: 6 in, 1 out]
                n171 = Unflatten From String(type="", binary string=w501, data includes array or string size? (T)=TRUE, error in (no error)=w503) -> (value=w500:string, error out=w502:errorcluster)  [unwired: 1 in, 1 out]
              }
            }
            n172 = call "MD5.vi"("Message String"=w482) -> ("MD5 (16-bytes)"=w480:string)  [unwired: 9 in, 1 out]
            n173 = Bundle By Name(cluster=w494, "Diagram (md5)"=w480) -> (w481:T5)
          }
          frame "calc_new_password" {
            w531 = ""  # New Password ("")
            # "BDPW data"
            # "LVSR data"
            # "Replace BDPW"
            # "Hash2 (MD5)"
            # "Diagram (MD5)"
            # "Hash1 (MD5)"
            # "New Password (MD5)\nLIBN (delimiter ':')\nLVSR\n<Salt (MD5)>"
            # "Pwrd (MD5)"
            # "Pwrd (MD5)\nHash1 (MD5)\nHash2 (MD5)"
            n174 = Unbundle By Name(w530) -> ("Owning Libs (':')"=w529:string, "Pswrd Salt (md5)"=w528:string, "Diagram (md5)"=w527:string)
            n175 = Unbundle By Name(w526) -> ("BDPW"=w525:i32, "LVSR"=w522:i32)
            n176 = Index Array(array=w524, index #1=w525, index #2=w522) -> (element #1=w523:T2, element #2=w521:T2)
            n177 = Unbundle By Name(w521) -> ("Data"=w519:string)
            n178 = call "MD5.vi"("Message String"=w531) -> ("MD5 (16-bytes)"=w534:string)  [unwired: 9 in, 1 out]
            n179 = Concatenate Strings(w534, w529, w519, w528) -> (w536:string)
            n180 = call "MD5.vi"("Message String"=w536) -> ("MD5 (16-bytes)"=w533:string)  [unwired: 9 in, 1 out]
            n181 = Concatenate Strings(w533, w527) -> (w535:string)
            n182 = call "MD5.vi"("Message String"=w535) -> ("MD5 (16-bytes)"=w532:string)  [unwired: 9 in, 1 out]
            n183 = Unbundle By Name(w523) -> ("Offset"=w516:u32, "Data"=w520:string)
            n184 = Concatenate Strings(w534, w533, w532) -> (w537:string)
            n185 = Replace Substring(3:0 ("offset (0)"), 4:w537, 5:w520) -> (1:w517:string)  [unwired: 1 in, 1 out]
            n186 = Bundle By Name(cluster=w530, "BDPW Offset"=w516, "New BDPW"=w517) -> (w518:T5)
            n187 = Select(t="overwrite_vi", s=w514, f="new_vi") -> (s? t:f=w513:string)
          }
          frame "new_vi" {
            # "Copy source VI and replace the BDPW block data, \nthen use VI scripting to create a clone of the VI\nto open in a new application context, finally delete\nthe temporary file."
            n188 = Unbundle By Name(w550) -> ("BDPW Offset"=w548:u32, "New BDPW"=w549:string)
            n189 = Read from Binary File(5:u8 0 ("unsigned byte array"), 8:w546, 10:-1 ("count (1)"), 11:w543) -> (0:w573:errorcluster, 2:w569:u8[], 3:w572:refnum<file>)  [unwired: 2 in, 1 out]
            n190 = String To Byte Array(string=w549) -> (unsigned byte array=w568:u8[])
            n191 = Close File(refnum=w572, error in=w573) -> (error out=w553:errorcluster)  [unwired: 1 out]
            n192 = Replace Array Subset(array=w569, new element=w568, index=w548) -> (w559:u8[])
            n193 = call <vilib>:"Get File Extension.vi"("error in (no error)"=w553, "file"=w543) -> ("error out"=w555:errorcluster, "filename without extension"=w554:string)  [unwired: 5 in, 3 out]
            n194 = call <vilib>:"Generate Temporary File Path.vi"("error in (no error)"=w555, "Temporary File Extension (tmp)"=w554) -> ("error out"=w552:errorcluster, "Unique Temporary File Path"=w560:path)  [unwired: 8 in]
            n195 = Open/Create/Replace File(file path (use dialog)=w560, error in=w552, operation (0:open)=T3."replace or create", access (0:read/write)=enum16{"read/write", "read-only", "write-only"}."write-only") -> (refnum out=w562:refnum<file>, error out=w565:errorcluster)  [unwired: 3 out]
            n196 = Write to Binary File(file (use dialog)=w562, data=w559, error in=w565, 5:FALSE ("prepend array or string size? (T)")) -> (refnum out=w564:refnum<file>, error out=w563:errorcluster)  [unwired: 2 in, 1 out]
            n197 = Close File(refnum=w564, error in=w563) -> (path=w557:path, error out=w558:errorcluster)
            n198 = case shown="No Error" w558 {
              selector: w558 -> [w594 w596]
              tunnel: [w595 w596] -> w556
              tunnel: w557 -> [w593 _]
              tunnel: w544 -> [w584 _]
              tunnel: w543 -> [w583 _]
              frame No Error {
                w581 = FALSE ("Save a Copy")
                n199 = New VI(8:w594, 10:w593) -> (0:w590:errorcluster, 3:w591:refnum<vi>)  [unwired: 5 in]
                n200 = Strip Path(path=w583) -> (name=w582:string)  [unwired: 1 out]
                n201 = Build Path(base path=w584, name or relative path=w582) -> (appended path=w585:path)
                n202 = invoke class="VI" method="Lock State.Set"(reference=w591, error in=w590, "lockState"=T7."Not Locked" ("Lock State")) -> (reference out=w589:refnum<vi>, error out=w588:errorcluster)  [unwired: 4 in, 5 out]
                n203 = invoke class="VI" method="Save.Instrument"(reference=w589, error in=w588, "Path to saved file"=w585, "Save a Copy"=w581, "Without Diagram"=w581) -> (reference out=w587:refnum<vi>, error out=w586:errorcluster)  [unwired: 1 in, 4 out]
                n204 = Close Reference(reference=w587, error in (no error)=w586) -> (error out=w595:errorcluster)
              }
              frame Error {
              }
            }
            n205 = flat-sequence {
              tunnel: w557 -> [w580]
              tunnel: [w579] -> w547
              tunnel: w556 -> [w579]
              frame #0 {
                n206 = Delete(path (use dialog)=w580) -> ()  [unwired: 4 in, 3 out]
              }
            }
          }
          frame "overwrite_vi" {
            # "Replace the BDPW block data in the existing VI, unlock and save"
            n207 = Unbundle By Name(w603) -> ("BDPW Offset"=w601:u32, "New BDPW"=w602:string)
            n208 = Read from Binary File(5:u8 0 ("unsigned byte array"), 8:w600, 10:-1 ("count (1)"), 11:w597) -> (0:w621:errorcluster, 2:w617:u8[], 3:w620:refnum<file>)  [unwired: 2 in, 1 out]
            n209 = String To Byte Array(string=w602) -> (unsigned byte array=w616:u8[])
            n210 = Close File(refnum=w620, error in=w621) -> (error out=w598:errorcluster)  [unwired: 1 out]
            n211 = Replace Array Subset(array=w617, new element=w616, index=w601) -> (w608:u8[])
            n212 = Open/Create/Replace File(file path (use dialog)=w597, error in=w598, operation (0:open)=T3."replace or create", access (0:read/write)=enum16{"read/write", "read-only", "write-only"}."write-only") -> (refnum out=w610:refnum<file>, error out=w613:errorcluster)  [unwired: 3 out]
            n213 = Write to Binary File(file (use dialog)=w610, data=w608, error in=w613, 5:FALSE ("prepend array or string size? (T)")) -> (refnum out=w612:refnum<file>, error out=w611:errorcluster)  [unwired: 2 in, 1 out]
            n214 = Close File(refnum=w612, error in=w611) -> (path=w606:path, error out=w607:errorcluster)
            n215 = case shown="No Error" w607 {
              selector: w607 -> [w629 w638]
              tunnel: [w637 w638] -> w605
              tunnel: w606 -> [w630 _]
              frame No Error {
                w631 = FALSE ("Save a Copy")
                n216 = Open VI Reference(vi path=w630, error in (no error)=w629) -> (vi reference=w628:refnum<vi>, error out=w627:errorcluster)  [unwired: 4 in]
                n217 = invoke class="VI" method="Lock State.Set"(reference=w628, error in=w627, "lockState"=T7."Not Locked" ("Lock State")) -> (reference out=w635:refnum<vi>, error out=w634:errorcluster)  [unwired: 4 in, 5 out]
                n218 = invoke class="VI" method="Save.Instrument"(reference=w635, error in=w634, "Save a Copy"=w631, "Without Diagram"=w631) -> (reference out=w633:refnum<vi>, error out=w632:errorcluster)  [unwired: 2 in, 4 out]
                n219 = Close Reference(reference=w633, error in (no error)=w632) -> (error out=w637:errorcluster)
              }
              frame Error {
              }
            }
          }
        }
        n220 = Or(x=w26, y=w23) -> (x .or. y?=w25:bool)
      }
    }
    frame Error {
    }
  }
  "error out" <- w4
